vi "MultiLag.vi"(8 "ErrI":errorcluster) -> (0 "ErrO":errorcluster)   [LabVIEW 2020]
doc: "Use this template to create a dialog box with event handling."
panel:
  in  "Lang":u16(ring) caption="Language" items=["English.ini", "简体中文.ini"]
  in  "Listbox":i32(listbox)
  in  "Tab Control":enum32{"Page 1", "Page 2"}(tab) caption="选项卡"
  in  "String":string
  in  "Numeric":dbl
  in  "Exit":bool
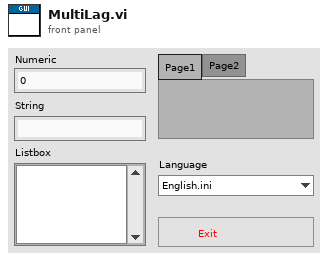
[diagram p1: front panel]
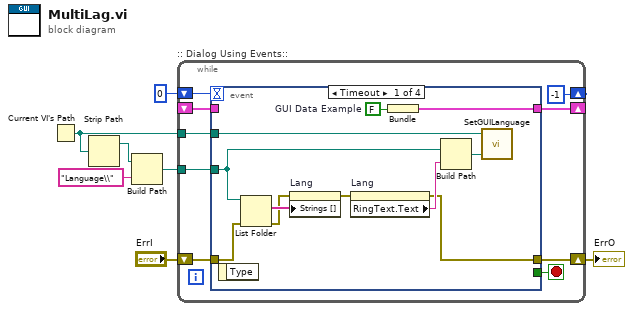
[diagram p0: block diagram]
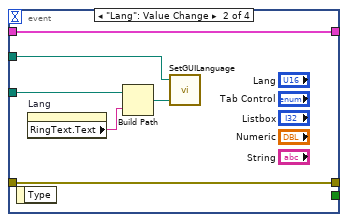
[diagram p2: hidden frame]
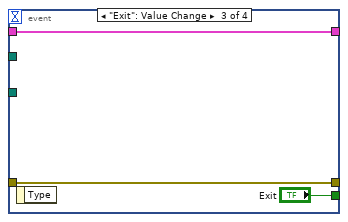
[diagram p3: hidden frame]
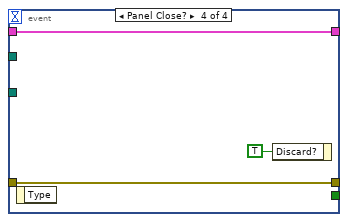
[diagram p4: hidden frame]
diagram:
  n1 = Current VI's Path() -> (path=w1:path)
  n2 = Strip Path(path=w1) -> (stripped path=w4:path)  [unwired: 1 out]
  n3 = Build Path(base path=w4, name or relative path="Language\\" ("string")) -> (appended path=w2:path)
  n4 = while ":: Dialog Using Events::" {
    shift-right: [w13] -> w6
    shift-left: "ErrI" -> [w12]
    shift-right: [w15] -> _
    shift-left: _ -> [w14]
    shift-right: [-1] -> _
    shift-left: 0 -> [w10]
    tunnel: w2 -> [w9]
    tunnel: w1 -> [w8]
    stop <- w16 stop-if-true
    n5 = event shown="[0] Timeout" {
      selector: _ -> [_ _ _ _]
      dyn-events: _ -> [_ _ _ _]
      timeout: w10 -> [_ _ _ _]
      tunnel: [_ _ "Exit" _] -> w16
      tunnel: w12 -> [w18 w33 w35 w39]
      tunnel: [w17 w33 w35 w39] -> w13
      tunnel: [w26 w32 w36 w37] -> w15
      tunnel: w14 -> [_ w32 w36 w37]
      tunnel: w9 -> [w22 w31 _ _]
      tunnel: w8 -> [w21 w28 _ _]
      event Timeout {
        w27 = FALSE  # GUI Data Example
        n6 = event-data() -> ()  [unwired: 2 out]
        n7 = List Folder(path=w22, error in=w18) -> (filenames=w25:string[], error out=w20:errorcluster)  [unwired: 2 in, 2 out]
        n8 = property on="Lang" class="Ring (strict)"(error in=w20, "Strings []"=w25) -> (error out=w19:errorcluster)  [unwired: 1 in, 1 out]
        n9 = property on="Lang" class="Ring (strict)"(error in=w19) -> (error out=w17:errorcluster, "RingText.Text"=w24:string)  [unwired: 1 in, 1 out]
        n10 = Bundle("GUI Data Example"=w27) -> (w26:cluster{"GUI Data Example":bool})  [unwired: 1 in]
        n11 = Build Path(base path=w22, name or relative path=w24) -> (appended path=w23:path)
        n12 = call "SetGUILanguage.vi"("Lang file path"=w23, "viPath"=w21) -> ()  [unwired: 1 out]
      }
      event "Lang": Value Change {
        n13 = event-data() -> ()  [unwired: 2 out]
        n14 = property on="Lang" class="Ring (strict)"() -> ("RingText.Text"=w30:string)  [unwired: 2 in, 2 out]
        n15 = Build Path(base path=w31, name or relative path=w30) -> (appended path=w29:path)
        n16 = call "SetGUILanguage.vi"("Lang file path"=w29, "viPath"=w28) -> ()  [unwired: 1 out]
      }
      event "Exit": Value Change {
        n17 = event-data() -> ()  [unwired: 2 out]
      }
      event Panel Close? {
        n18 = event-data() -> ()  [unwired: 2 out]
        n19 = event-data("Discard?"=TRUE ("Cancelled?")) -> ()  [unwired: 1 in, 1 out]
      }
    }
  }
  "ErrO" <- w6
